vi "InsertMoney.vi"(8 "error in (no error)":errorcluster, 11 "object in":refnum<class "HasMoneyState.lvclass">) -> (0 "error out":errorcluster, 3 "object out":refnum<class "State.lvclass">)   [LabVIEW 2020, in "HasMoneyState.lvclass"]
uses:
  HasMoneyState.lvclass
  C:/Projects/DesignPatterns/StatePattern/State_class/State.lvclass
  State_class/State.lvclass
  <userlib>/_LabVIEWCommon/LcDialogs/LcDialog_AutoSizeDialog_Font.ctl
  HasMoneyState.lvclass/HasMoneyState.ctl
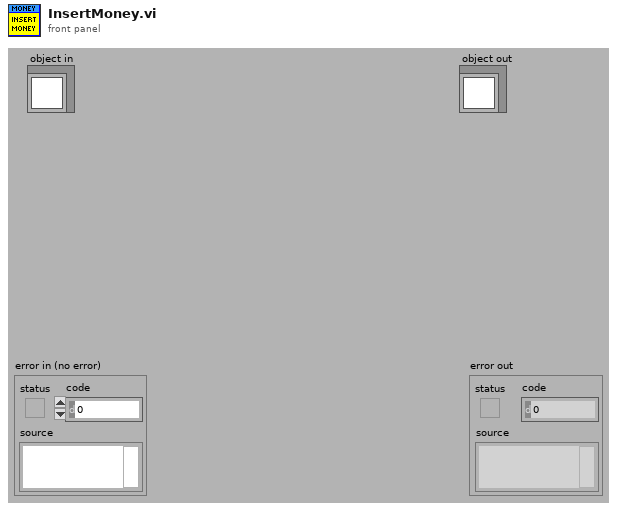
[diagram p1: front panel]
types:
  T1 = typedef "LcDialog_AutoSizeDialog_Font.ctl" = cluster{"Size":u32, "Bold":bool, "Color":u32}
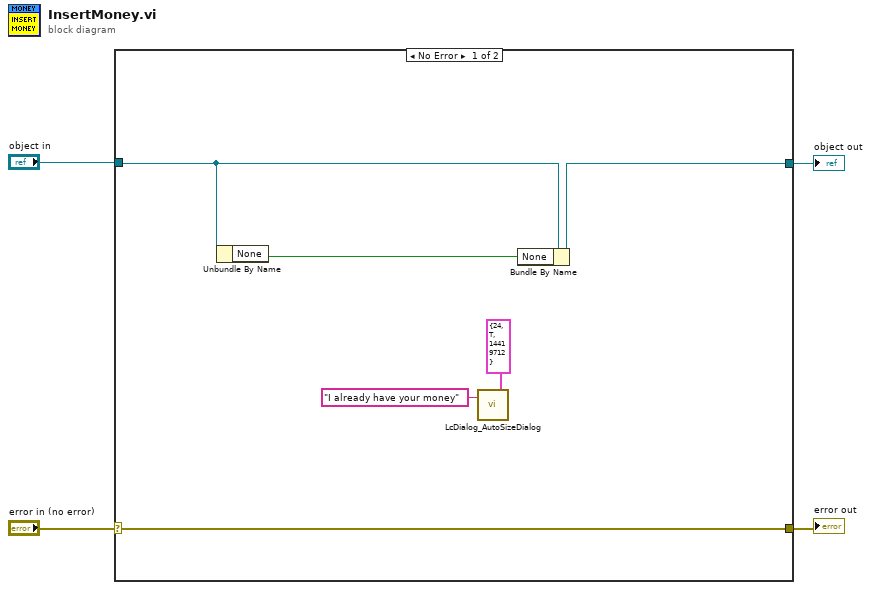
[diagram p0: block diagram]
diagram:
  n1 = case shown="No Error" "error in (no error)" {
    selector: "error in (no error)" -> [w9 w12]
    tunnel: [w9 w12] -> w3
    tunnel: [w7 w11] -> w1
    tunnel: "object in" -> [w8 w11]
    frame No Error {
      n2 = Unbundle By Name(w8) -> ("None"=w10:bool)
      n3 = call <userlib>:"LcDialog_AutoSizeDialog.vi"("TextIn"="I already have your money", "FontSettings"=T1 {"Size"=24, "Bold"=TRUE, "Color"=14419712}) -> ()  [unwired: 13 in, 5 out]
      n4 = Bundle By Name(cluster=w8, "None"=w10) -> (w7:refnum<class "HasMoneyState.lvclass">)
    }
    frame Error {
    }
  }
  "error out" <- w3
  "object out" <- w1
